vi "Write Serial Session.vi"(8 "error in (no error)":errorcluster, 10 "Session Handle":T1, 11 "PPT in":refnum<class "PPT.lvclass">) -> (0 "error out":errorcluster, 3 "PPT out":refnum<class "PPT.lvclass">)   [LabVIEW 2014, in "PPT Library.lvlib" / "PPT.lvclass"]
uses:
  PPT.lvclass
  <userlib>/_Session Fwk/Typedefs/Session Handle.ctl
  <userlib>/_Session Fwk/Session - Root.lvclass
  PPT.lvclass/PPT.ctl
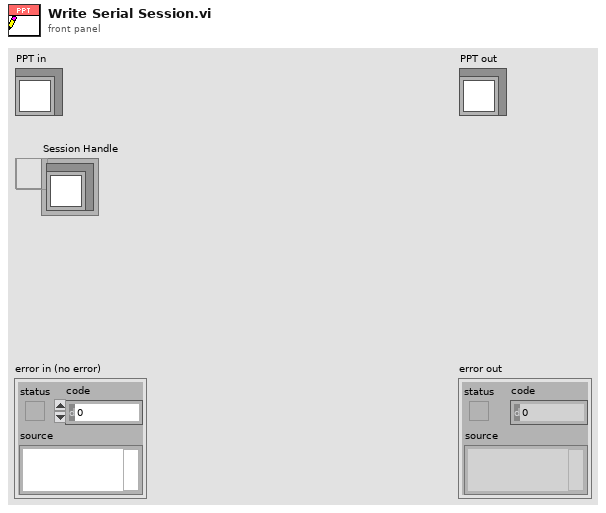
[diagram p1: front panel]
types:
  T1 = typedef "Session - Root.lvclass/Session Handle.ctl" = refnum<data-value>
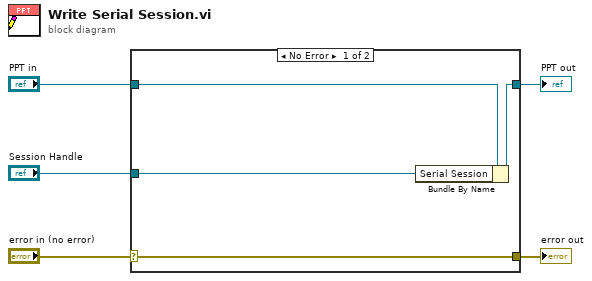
[diagram p0: block diagram]
diagram:
  n1 = case shown="No Error" "error in (no error)" {
    selector: "error in (no error)" -> [w9 w10]
    tunnel: [w9 w10] -> w4
    tunnel: [w7 w11] -> w2
    tunnel: "PPT in" -> [w8 w11]
    tunnel: "Session Handle" -> [w6 _]
    frame No Error {
      n2 = Bundle By Name(cluster=w8, "Serial Session"=w6) -> (w7:refnum<class "PPT.lvclass">)
    }
    frame Error {
    }
  }
  "error out" <- w4
  "PPT out" <- w2
